vi "Configure Step Cycle.vi"(0 "VISA resource name":refnum<visa-resource-name>, 5 "Step Cycle (1)":i32=1 min=0 max=9999 step=1, 11 "error in (no error)":errorcluster) -> (4 "VISA resource name out":refnum<visa-resource-name>, 15 "error out":errorcluster)   [LabVIEW 2014, in "eec 6700.lvlib"]
doc: "Sets the <B>Step Cycle</B> of the active step in the current Memory location (Use \"Configure Memory.vi\" to select the desired memory)\n\n<B>Range</B> : 0~9999 ,0=Continue,1=Off\n\nThe step cycle parameter setting configures the number of looping cycles for a particular step. For example if the operator would like to have a step repeat five times the step cycle would be programmed to five."
uses:
  <instrlib>/eec 6700/eec 6700.lvlib
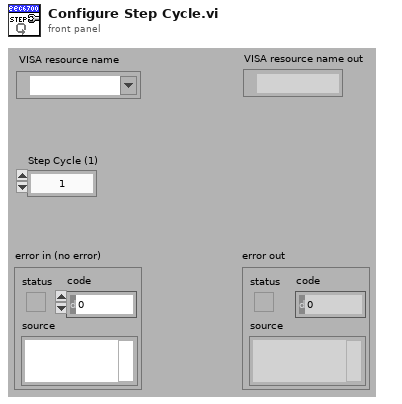
[diagram p1: front panel]
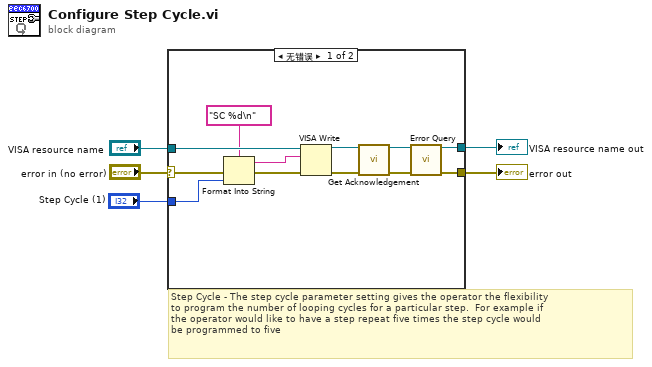
[diagram p0: block diagram]
diagram:
  # "Step Cycle - The step cycle parameter setting gives the operator the flexibility \nto program the number of looping cycles for a particular step.  For example if \nthe operator would like to have a step repeat five times the step cycle would \nbe programmed to five"
  n1 = case shown="无错误" "error in (no error)" {
    selector: "error in (no error)" -> [w11 w19]
    tunnel: "VISA resource name" -> [w17 w18]
    tunnel: [w13 w18] -> w4
    tunnel: [w12 w19] -> w3
    tunnel: "Step Cycle (1)" -> [w16 _]
    frame No Error {
      n2 = Format Into String(format string="SC %d\n" ("Command"), error in=w11, w16) -> (resulting string=w15:string, error out=w10:errorcluster)  [unwired: 1 in]
      n3 = VISA Write(VISA resource name=w17, write buffer=w15, error in (no error)=w10) -> (VISA resource name out=w6:refnum<visa-resource-name>, error out=w9:errorcluster)  [unwired: 1 out]
      n4 = call <instrlib>:"Get Acknowledgement.vi"("VISA resource name"=w6, "error in (no error)"=w9) -> ("VISA resource name out"=w7:refnum<visa-resource-name>, "error out"=w8:errorcluster)  [unwired: 12 in]
      n5 = call <instrlib>:"Error Query.vi"("VISA resource name"=w7, "error in (no error)"=w8) -> ("VISA resource name out"=w13:refnum<visa-resource-name>, "error out"=w12:errorcluster)  [unwired: 10 in, 2 out]
    }
    frame Error {
    }
  }
  "error out" <- w3
  "VISA resource name out" <- w4
